vi "20TILM_Queue_Commands.vi"(1 "20TILM Control (in)":T1, 2 "ILM Queue":refnum<queue>) -> (0 "20TILM Control (out)":T1)   [LabVIEW 2019]
uses:
  Gustav/20TILM_Control.ctl
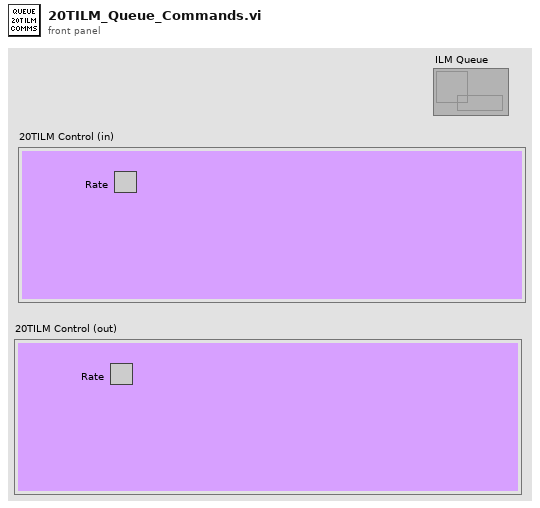
[diagram p1: front panel]
types:
  T1 = typedef "20TILM_Control.ctl" = cluster{"Rate":bool}
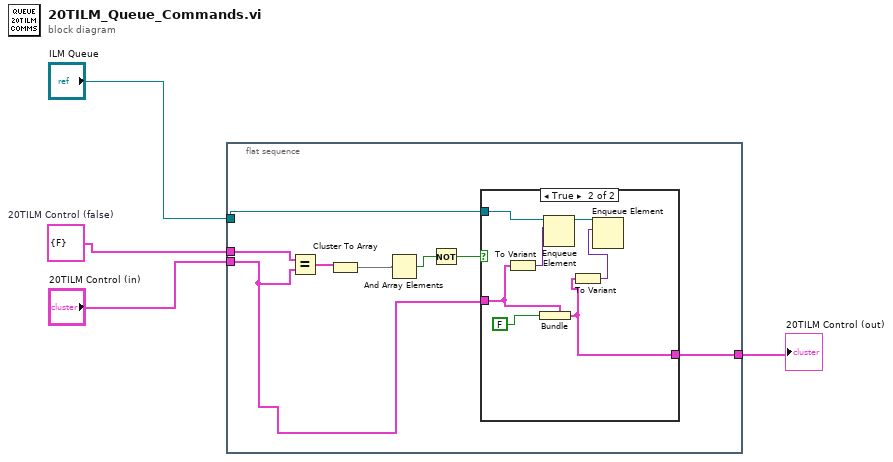
[diagram p0: block diagram]
diagram:
  w1 = T1 {"Rate"=FALSE}  # 20TILM Control (false)
  n1 = flat-sequence {
    tunnel: "ILM Queue" -> [w12]
    tunnel: "20TILM Control (in)" -> [w5]
    tunnel: w1 -> [w6]
    tunnel: [w7] -> w3
    frame #0 {
      n2 = Equal?(x=w6, y=w5) -> (x = y?=w8:T1)
      n3 = Cluster To Array(cluster=w8) -> (array=w11:bool[])
      n4 = And Array Elements(Boolean array=w11) -> (logical AND=w10:bool)
      n5 = Not(x=w10) -> (.not. x?=w9:bool)
      n6 = case shown="True" w9 {
        tunnel: w12 -> [_ w20]
        tunnel: w5 -> [w13 w16]
        tunnel: [w13 w15] -> w7
        frame False {
        }
        frame True {
          n7 = To Variant(anything=w16) -> (Variant=w19:variant)
          n8 = Bundle ("Bündeln")(cluster=w16, "Rate"=FALSE) -> (w15:T1)
          n9 = Enqueue Element(queue=w20, element=w19) -> (queue out=w18:refnum<queue>)  [unwired: 2 in, 2 out]
          n10 = To Variant(anything=w15) -> (Variant=w17:variant)
          n11 = Enqueue Element(queue=w18, element=w17) -> ()  [unwired: 2 in, 3 out]
        }
      }
    }
  }
  "20TILM Control (out)" <- w3
